vi "PriorityQueue.vi"() -> ()   [LabVIEW 2019]
uses:
  <userlib>/National Instruments/Priority Queue/Data.ctl
  <userlib>/National Instruments/Priority Queue/Priority Queue.lvclass
panel:
  out "Actual Array":T1[](array[typedef])
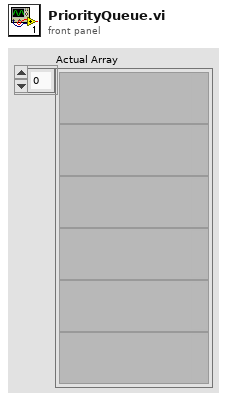
[diagram p1: front panel]
types:
  T1 = typedef "Priority Queue.lvclass/Data.ctl" = variant
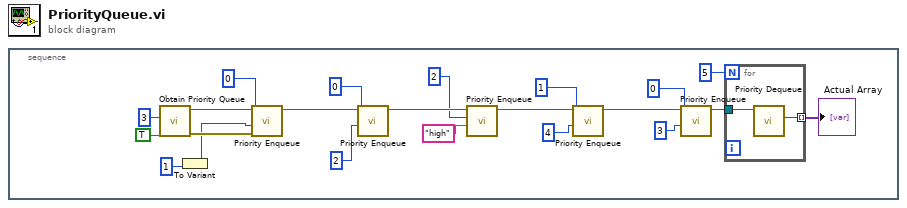
[diagram p0: block diagram]
diagram:
  n1 = stacked-sequence {
    frame #0 {
      n2 = call <userlib>:"Obtain Priority Queue.vi"("create if not found? (T)"=TRUE, "# of priorities"=3) -> ("error out"=w14:errorcluster, "Priority Queue"=w22:refnum<class "Priority Queue.lvclass">)  [unwired: 7 in, 1 out]
      n3 = To Variant(anything=1) -> (Variant=w5:variant)
      n4 = call <userlib>:"Priority Enqueue.vi"("error in (no error)"=w14, "element"=w5, "priority"=0, "Priority Queue in"=w22) -> ("Priority Queue out"=w21:refnum<class "Priority Queue.lvclass">)  [unwired: 6 in, 1 out]
      n5 = call <userlib>:"Priority Enqueue.vi"("element"=2, "priority"=0, "Priority Queue in"=w21) -> ("Priority Queue out"=w20:refnum<class "Priority Queue.lvclass">)  [unwired: 7 in, 1 out]
      n6 = call <userlib>:"Priority Enqueue.vi"("element"="high", "priority"=2, "Priority Queue in"=w20) -> ("Priority Queue out"=w19:refnum<class "Priority Queue.lvclass">)  [unwired: 7 in, 1 out]
      n7 = call <userlib>:"Priority Enqueue.vi"("element"=4, "priority"=1, "Priority Queue in"=w19) -> ("Priority Queue out"=w16:refnum<class "Priority Queue.lvclass">)  [unwired: 7 in, 1 out]
      n8 = call <userlib>:"Priority Enqueue.vi"("element"=3, "priority"=0, "Priority Queue in"=w16) -> ("Priority Queue out"=w15:refnum<class "Priority Queue.lvclass">)  [unwired: 7 in, 1 out]
      n9 = for {
        N: 5 -> [_]
        tunnel: w15 -> [w24]
        tunnel: [w23] -> w17 mode=indexing
        n10 = call <userlib>:"Priority Dequeue.vi"("Priority Queue in"=w24) -> ("element"=w23:T1)  [unwired: 7 in, 3 out]
      }
      "Actual Array" <- w17
    }
  }
